vi "Value Changed.vi"(7 "Numeric":i32) -> (8 "Changed":bool)   [LabVIEW 2015]
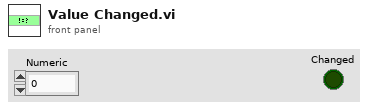
[diagram p1: front panel]
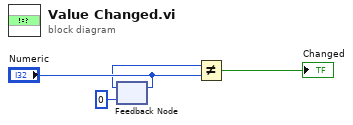
[diagram p0: block diagram]
diagram:
  n1 = feedback-in #1("Numeric") -> ()
  n2 = feedback #1(0 ("Numeric")) -> (w2:i32)
  n3 = Not Equal?(x=w2, y="Numeric") -> (x != y?=→"Changed":bool)
